vi "FTW-File-CreateDirectory.vi"(0 "Directory to Create":path, 11 "error in":errorcluster) -> (4 "Created Directory":path, 15 "error out":errorcluster)   [LabVIEW 2014]
panel:
  # "Inputs"
  # "Outputs"
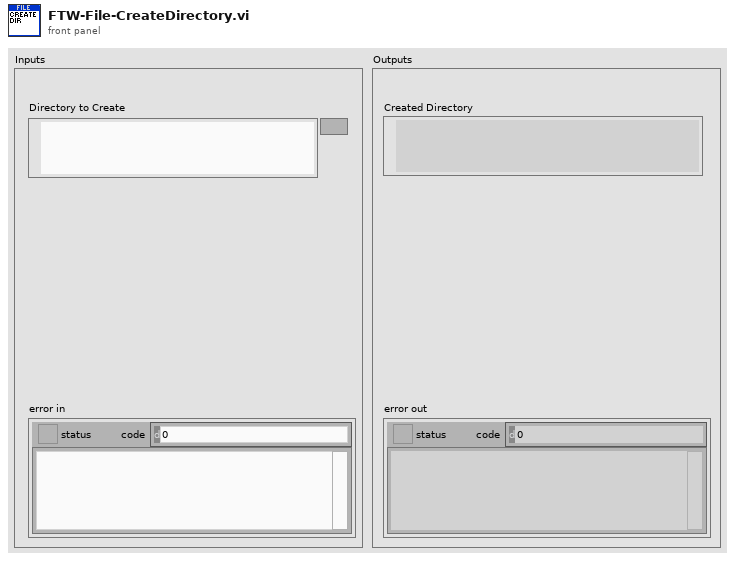
[diagram p1: front panel]
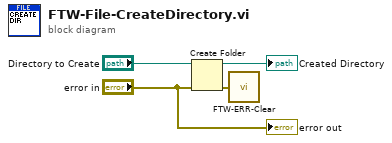
[diagram p0: block diagram]
diagram:
  n1 = Create Folder(path (use dialog)="Directory to Create", error in="error in") -> (created path=→"Created Directory":path, error out=w1:errorcluster)  [unwired: 1 in, 1 out]
  n2 = call "FTW-ERR-Clear.vi"("error to snuff"=w1) -> ()  [unwired: 1 out]
  "error out" <- "error in"
